vi "Read Character.vi"(8 "error in (no error)":errorcluster, 11 "Character in":refnum<class "Character.lvclass">) -> (0 "error out":errorcluster, 2 "Character":u8 format="%.0x", 3 "Character out":refnum<class "Character.lvclass">)   [LabVIEW 2016, in "Character.lvclass"]
uses:
  Character.lvclass
  Character.lvclass/Character.ctl
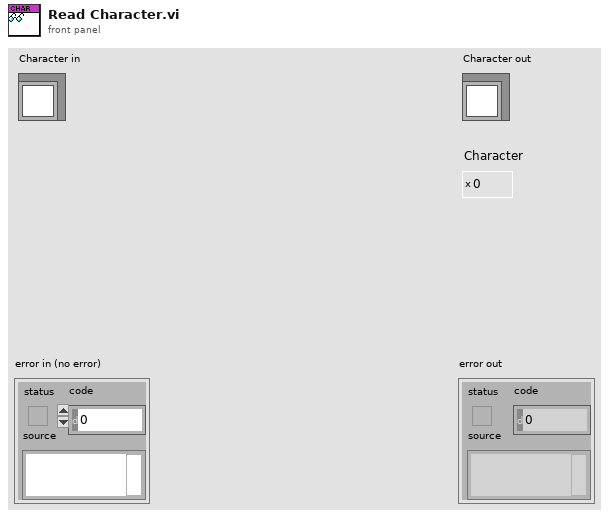
[diagram p1: front panel]
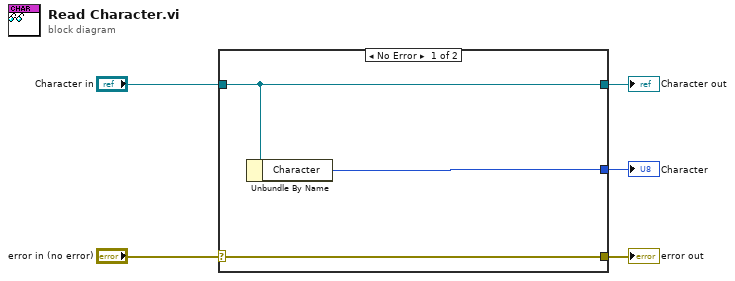
[diagram p0: block diagram]
diagram:
  n1 = case shown="No Error" "error in (no error)" {
    selector: "error in (no error)" -> [w8 w9]
    tunnel: [w8 w9] -> w4
    tunnel: [w7 w10] -> w2
    tunnel: "Character in" -> [w7 w10]
    tunnel: [w6 _] -> w1
    frame No Error {
      n2 = Unbundle By Name(w7) -> ("Character"=w6:u8)
    }
    frame Error {
    }
  }
  "error out" <- w4
  "Character out" <- w2
  "Character" <- w1
